vi "InsertIntoString.vi"(10 "Items":string[](array[string])=["C1", "C2", "C3"], 11 "Table Name":string="temp") -> (3 "Insert Into String":string)   [LabVIEW 2015, in "DBToolkit.lvlib"]
uses:
  DBToolkit.lvlib
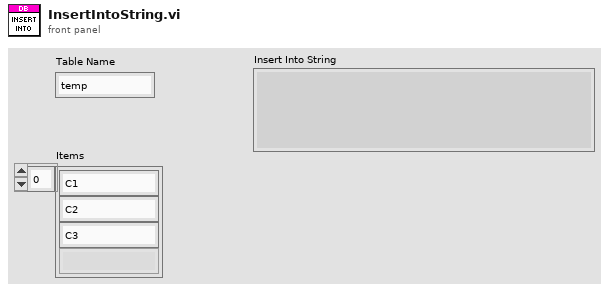
[diagram p1: front panel]
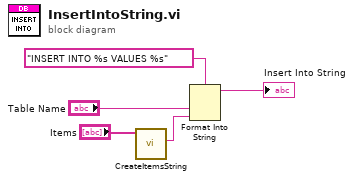
[diagram p0: block diagram]
diagram:
  n1 = call "CreateItemsString.vi"("Items"="Items") -> ("Items for INSERT"=w2:string)  [unwired: 8 in, 2 out]
  n2 = Format Into String(format string="INSERT INTO %s VALUES %s" ("string"), "Table Name", w2) -> (resulting string=→"Insert Into String":string)  [unwired: 2 in, 1 out]
